vi "getBorderNum.vi"(0 "Refnum in":T1, 2 "Cut Limit":dbl format="%#_13g", 5 "Bounding Box":cluster{"x":sgl, "y":sgl}[][](array[cluster]), 7 "Position":sgl[][](array[numeric]), 9 "Angle":sgl[](array[numeric]), 11 "error in (no error)":errorcluster, 12 "Step":sgl=0.29742944, 13 "Origin Pixel":dbl[](array[numeric])) -> (4 "Refnum out":T1, 8 "Data Pieces":T3(array[cluster]) {"ROI Números"."Contours"."Type" items=["No Selection", "Point", "Line", "Rectangle", "Oval", "Polygon", "Freehand Region", "Annulus", "Unused2", "Unused3", "Broken Line", "Freehand Line", "Rotated Rectangle"]}, 15 "error out":errorcluster)   [LabVIEW 2016]
uses:
  <vilib>/vision/Image Controls.llb/IMAQ Image.ctl
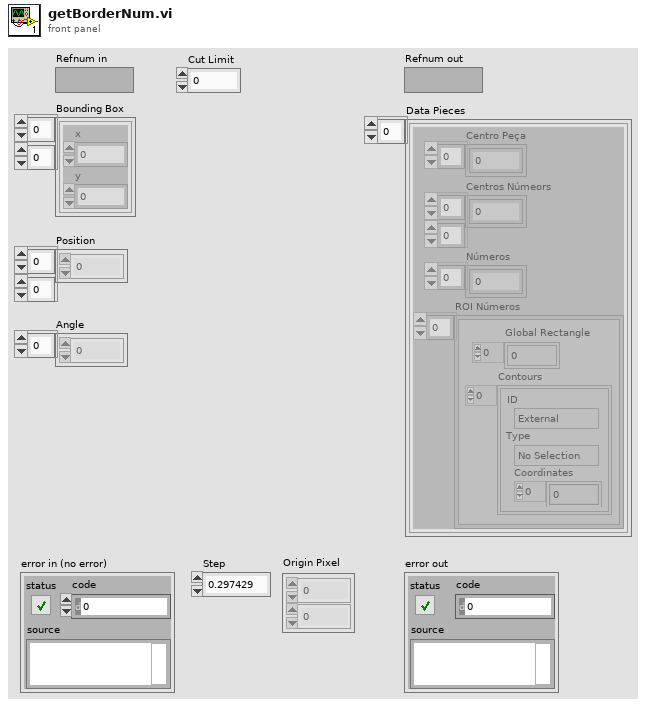
[diagram p1: front panel]
types:
  T1 = typedef "IMAQ Image.ctl" = refnum<image>
  T2 = typedef "ROI Descriptor" = cluster{"Global Rectangle":i32[], "Contours":cluster{"ID":enum32{"External", "Internal"}, "Type":u32, "Coordinates":i32[]}[]}
  T3 = cluster{"Centro Peça":dbl[], "Centros Númeors":dbl[][], "Números":u8[], "ROI Números":T2[]}[]
  T4 = cluster{"Centro Peça":dbl[], "Centros Númeors":dbl[][], "Números":u8[], "ROI Números":T2[]}
  T5 = typedef "IMAQ Rectangle" = cluster{"Left":i32, "Top":i32, "Right":i32, "Bottom":i32, "Rotation":dbl}
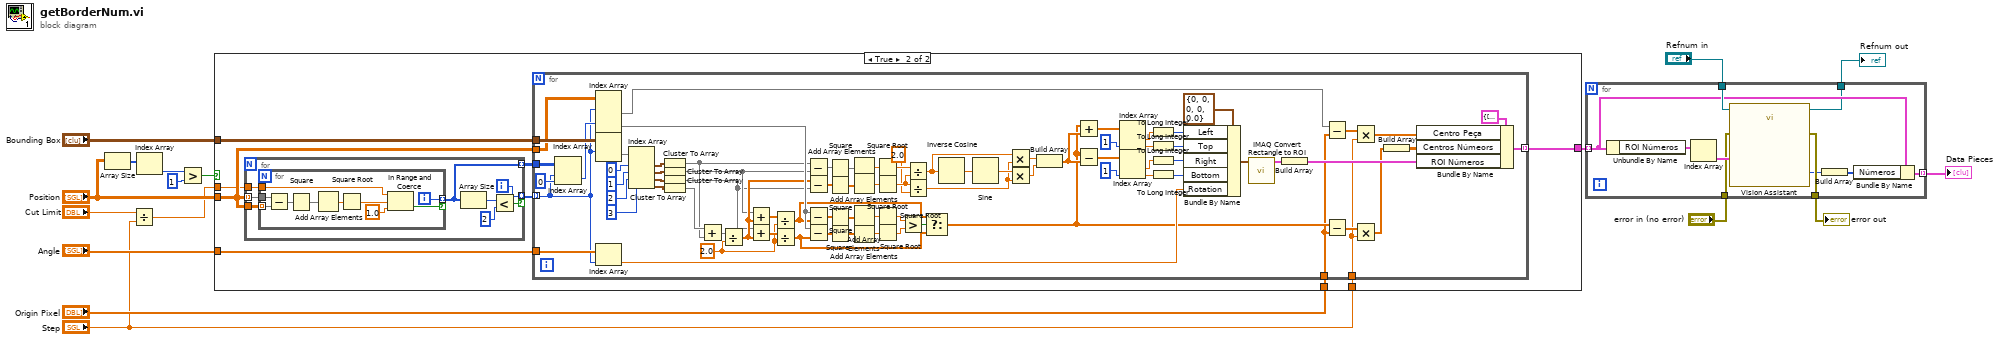
[diagram p0: block diagram]
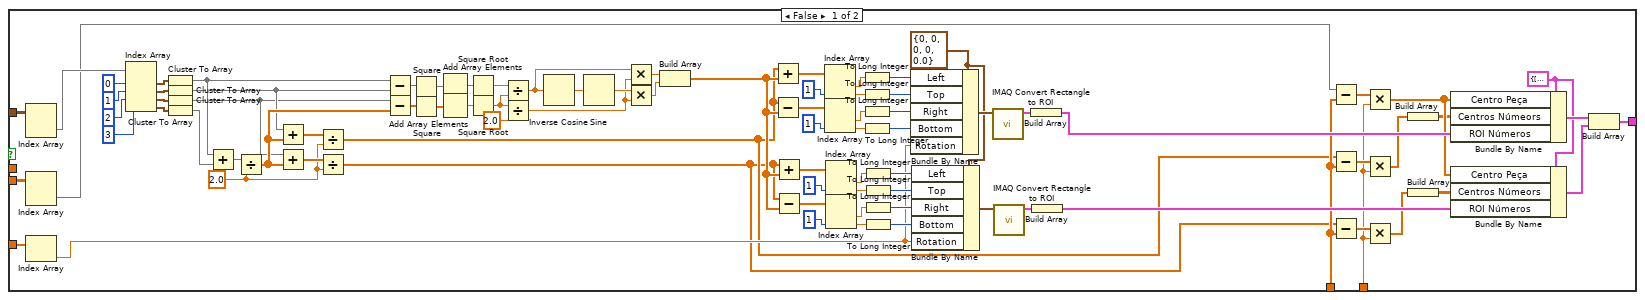
[diagram p2: hidden frame]
diagram:
  n1 = Array Size(array="Position") -> (size(s)=w7:i32[])
  n2 = Divide(x="Cut Limit", y="Step") -> (x/y=w3:dbl)
  n3 = Index Array(array=w7) -> (element=w8:i32)  [unwired: 1 in]
  n4 = Greater?(x=w8, y=1) -> (0:w6:bool)
  n5 = case shown="True" w6 {
    tunnel: "Bounding Box" -> [w103 w112]
    tunnel: "Position" -> [w102 w111]
    tunnel: "Angle" -> [w41 w109]
    tunnel: [w37 w107] -> w12
    tunnel: w3 -> [_ w106]
    tunnel: "Origin Pixel" -> [w24 w105]
    tunnel: "Step" -> [w25 w104]
    frame False {
      w36 = T4 {"Centro Peça"=[0.0, 0.0], "Centros Númeors"=[[0.0, 0.0], [0.0, 0.0]], "Números"=[0, 0], "ROI Números"=[]} ("Dados Peça")
      w42 = T5 {"Left"=0, "Top"=0, "Right"=0, "Bottom"=0, "Rotation"=0.0} ("Rectangle")
      w78 = 2.0 ("y")
      n6 = Index Array(array=w103) -> (element=w101:cluster{"x":sgl, "y":sgl}[])  [unwired: 2 in]
      n7 = Index Array(array=w102) -> (element=w29:sgl[])  [unwired: 2 in]
      n8 = Index Array(array=w41) -> (element=w40:sgl)  [unwired: 1 in]
      n9 = Index Array(array=w101, index #1=0 ("index"), index #2=1 ("index"), index #3=2 ("index"), index #4=3 ("index")) -> (element #1=w96:cluster{"x":sgl, "y":sgl}, element #2=w95:cluster{"x":sgl, "y":sgl}, element #3=w94:cluster{"x":sgl, "y":sgl}, element #4=w93:cluster{"x":sgl, "y":sgl})
      n10 = Cluster To Array(cluster=w96) -> (array=w84:sgl[])
      n11 = Cluster To Array(cluster=w95) -> (array=w82:sgl[])
      n12 = Cluster To Array(cluster=w94) -> (array=w81:sgl[])
      n13 = Cluster To Array(cluster=w93) -> (array=w89:sgl[])
      n14 = Add(x=w84, y=w89) -> (x+y=w88:sgl[])
      n15 = Divide(x=w88, y=w78) -> (x/y=w83:dbl[])
      n16 = Add(x=w82, y=w83) -> (x+y=w80:dbl[])
      n17 = Add(x=w81, y=w83) -> (x+y=w79:dbl[])
      n18 = Divide(x=w80, y=w78) -> (x/y=w23:dbl[])
      n19 = Divide(x=w79, y=w78) -> (x/y=w22:dbl[])
      n20 = Subtract(x=w84, y=w82) -> (x-y=w85:sgl[])
      n21 = Subtract(x=w81, y=w83) -> (x-y=w90:dbl[])
      n22 = Square(x=w85) -> (x^2=w87:sgl[])
      n23 = Square(x=w90) -> (x^2=w92:dbl[])
      n24 = Add Array Elements(numeric array=w87) -> (sum=w86:sgl)
      n25 = Add Array Elements(numeric array=w92) -> (sum=w91:dbl)
      n26 = Square Root(x=w86) -> (sqrt(x)=w77:sgl)
      n27 = Square Root(x=w91) -> (sqrt(x)=w76:dbl)
      n28 = Divide(x=w77, y=w76) -> (x/y=w70:dbl)
      n29 = Divide(x=w76, y=2.0) -> (x/y=w69:dbl)
      n30 = Inverse Cosine(1:w70) -> (0:w74:dbl)
      n31 = Sine(x=w74) -> (sin(x)=w73:dbl)
      n32 = Multiply(x=w70, y=w69) -> (x*y=w71:dbl)
      n33 = Multiply(x=w73, y=w69) -> (x*y=w72:dbl)
      n34 = Build Array(w71, w72) -> (w39:dbl[])
      n35 = Add(x=w23, y=w39) -> (x+y=w56:dbl[])
      n36 = Subtract(x=w23, y=w39) -> (x-y=w57:dbl[])
      n37 = Add(x=w22, y=w39) -> (x+y=w43:dbl[])
      n38 = Subtract(x=w22, y=w39) -> (x-y=w44:dbl[])
      n39 = Index Array(array=w56, index #2=1 ("index")) -> (element #1=w58:dbl, element #2=w59:dbl)  [unwired: 1 in]
      n40 = Index Array(array=w57, index #2=1 ("index")) -> (element #1=w60:dbl, element #2=w61:dbl)  [unwired: 1 in]
      n41 = Index Array(array=w43, index #2=1 ("index")) -> (element #1=w45:dbl, element #2=w46:dbl)  [unwired: 1 in]
      n42 = Index Array(array=w44, index #2=1 ("index")) -> (element #1=w47:dbl, element #2=w48:dbl)  [unwired: 1 in]
      n43 = To Long Integer(number=w58) -> (32bit integer=w65:i32)
      n44 = To Long Integer(number=w59) -> (32bit integer=w64:i32)
      n45 = To Long Integer(number=w60) -> (32bit integer=w63:i32)
      n46 = To Long Integer(number=w61) -> (32bit integer=w62:i32)
      n47 = To Long Integer(number=w45) -> (32bit integer=w52:i32)
      n48 = To Long Integer(number=w46) -> (32bit integer=w51:i32)
      n49 = To Long Integer(number=w47) -> (32bit integer=w50:i32)
      n50 = To Long Integer(number=w48) -> (32bit integer=w49:i32)
      n51 = Bundle By Name(cluster=w42, "Left"=w65, "Top"=w64, "Right"=w63, "Bottom"=w62, "Rotation"=w40) -> (w66:T5)
      n52 = Bundle By Name(cluster=w42, "Left"=w52, "Top"=w51, "Right"=w50, "Bottom"=w49, "Rotation"=w40) -> (w53:T5)
      n53 = call "IMAQ Convert Rectangle to ROI"("Rectangle"=w66) -> ("ROI Descriptor"=w35:T2)  [unwired: 8 in, 1 out]
      n54 = call "IMAQ Convert Rectangle to ROI"("Rectangle"=w53) -> ("ROI Descriptor"=w34:T2)  [unwired: 8 in, 1 out]
      n55 = Build Array(w35) -> (w32:T2[])
      n56 = Build Array(w34) -> (w33:T2[])
      n57 = Subtract(x=w29, y=w24) -> (x-y=w30:dbl[])
      n58 = Subtract(x=w23, y=w24) -> (x-y=w27:dbl[])
      n59 = Subtract(x=w22, y=w24) -> (x-y=w26:dbl[])
      n60 = Multiply(x=w30, y=w25) -> (x*y=w28:dbl[])
      n61 = Multiply(x=w27, y=w25) -> (x*y=w21:dbl[])
      n62 = Multiply(x=w26, y=w25) -> (x*y=w18:dbl[])
      n63 = Build Array(w21) -> (w20:dbl[][])
      n64 = Build Array(w18) -> (w19:dbl[][])
      n65 = Bundle By Name(cluster=w36, "Centro Peça"=w28, "Centros Númeors"=w20, "ROI Números"=w32) -> (w38:T4)
      n66 = Bundle By Name(cluster=w36, "Centro Peça"=w28, "Centros Númeors"=w19, "ROI Números"=w33) -> (w31:T4)
      n67 = Build Array(w38, w31) -> (w37:T3)
    }
    frame True {
      n68 = for {
        tunnel: w111 -> [w201] mode=indexing
        tunnel: w111 -> [w200]
        tunnel: [w199] -> w110 mode=indexing if=w196
        tunnel: [w195] -> w108 mode=indexing
        tunnel: w106 -> [w194]
        i -> [w199]
        n69 = for {
          tunnel: w201 -> [w211]
          tunnel: w200 -> [w207] mode=indexing
          tunnel: [w204] -> w195 mode=indexing if=w203
          tunnel: w194 -> [w202]
          i -> [w204]
          n70 = Subtract(x=w211, y=w207) -> (x-y=w210:sgl[])
          n71 = Square(x=w210) -> (x^2=w209:sgl[])
          n72 = Add Array Elements(numeric array=w209) -> (sum=w208:sgl)
          n73 = Square Root(x=w208) -> (sqrt(x)=w205:sgl)
          n74 = In Range and Coerce(upper limit=w202, x=w205, lower limit=1.0) -> (In Range?=w203:bool)  [unwired: 1 out]
        }
        n75 = Array Size(array=w195) -> (size(s)=w198:i32)
        n76 = Less?(x=w198, y=2) -> (x < y?=w196:bool)
      }
      n77 = for {
        tunnel: w112 -> [w193]
        tunnel: w111 -> [w191]
        tunnel: w110 -> [w153] mode=indexing
        tunnel: w109 -> [w179]
        tunnel: w108 -> [w176]
        tunnel: [w122] -> w107 mode=indexing
        tunnel: w105 -> [w114]
        tunnel: w104 -> [w113]
        w152 = 2.0 ("y")
        n78 = Index Array(array=w176, index (row)=w153, index (col)=0 ("disabled index (col)")) -> (element=w175:i32)
        n79 = Index Array(array=w191, index (row) #1=w153, index (row) #2=w175) -> (element #1=w121:sgl[], element #2=w154:sgl[])  [unwired: 2 in]
        n80 = Index Array(array=w193, index (row)=w153) -> (element=w192:cluster{"x":sgl, "y":sgl}[])  [unwired: 1 in]
        n81 = Index Array(array=w179, index=w153) -> (element=w178:sgl)
        n82 = Index Array(array=w192, index #1=0 ("index"), index #2=1 ("index"), index #3=2 ("index"), index #4=3 ("index")) -> (element #1=w189:cluster{"x":sgl, "y":sgl}, element #2=w190:cluster{"x":sgl, "y":sgl}, element #3=w188:cluster{"x":sgl, "y":sgl}, element #4=w171:cluster{"x":sgl, "y":sgl})
        n83 = Cluster To Array(cluster=w189) -> (array=w138:sgl[])
        n84 = Cluster To Array(cluster=w190) -> (array=w137:sgl[])
        n85 = Cluster To Array(cluster=w188) -> (array=w132:sgl[])
        n86 = Cluster To Array(cluster=w171) -> (array=w168:sgl[])
        n87 = Add(x=w168, y=w138) -> (x+y=w170:sgl[])
        n88 = Divide(x=w170, y=w152) -> (x/y=w143:dbl[])
        n89 = Add(x=w137, y=w143) -> (x+y=w142:dbl[])
        n90 = Add(x=w132, y=w143) -> (x+y=w167:dbl[])
        n91 = Divide(x=w142, y=w152) -> (x/y=w148:dbl[])
        n92 = Divide(x=w167, y=w152) -> (x/y=w147:dbl[])
        n93 = Subtract(x=w138, y=w137) -> (x-y=w139:sgl[])
        n94 = Subtract(x=w143, y=w132) -> (x-y=w146:dbl[])
        n95 = Subtract(x=w154, y=w148) -> (x-y=w166:dbl[])
        n96 = Subtract(x=w154, y=w147) -> (x-y=w155:dbl[])
        n97 = Square(x=w139) -> (x^2=w141:sgl[])
        n98 = Square(x=w146) -> (x^2=w144:dbl[])
        n99 = Square(x=w166) -> (x^2=w164:dbl[])
        n100 = Square(x=w155) -> (x^2=w157:dbl[])
        n101 = Add Array Elements(numeric array=w141) -> (sum=w140:sgl)
        n102 = Add Array Elements(numeric array=w144) -> (sum=w145:dbl)
        n103 = Add Array Elements(numeric array=w164) -> (sum=w165:dbl)
        n104 = Add Array Elements(numeric array=w157) -> (sum=w156:dbl)
        n105 = Square Root(x=w140) -> (sqrt(x)=w136:sgl)
        n106 = Square Root(x=w145) -> (sqrt(x)=w131:dbl)
        n107 = Square Root(x=w165) -> (sqrt(x)=w150:dbl)
        n108 = Square Root(x=w156) -> (sqrt(x)=w149:dbl)
        n109 = Greater?(x=w150, y=w149) -> (0:w151:bool)
        n110 = Divide(x=w136, y=w131) -> (x/y=w133:dbl)
        n111 = Divide(x=w131, y=2.0) -> (x/y=w129:dbl)
        n112 = Select(t=w148, s=w151, f=w147) -> (s? t:f=w115:dbl[])
        n113 = Inverse Cosine(1:w133) -> (0:w135:dbl)
        n114 = Sine(x=w135) -> (sin(x)=w134:dbl)
        n115 = Multiply(x=w133, y=w129) -> (x*y=w127:dbl)
        n116 = Multiply(x=w134, y=w129) -> (x*y=w128:dbl)
        n117 = Build Array(w127, w128) -> (w126:dbl[])
        n118 = Add(x=w115, y=w126) -> (x+y=w158:dbl[])
        n119 = Subtract(x=w115, y=w126) -> (x-y=w159:dbl[])
        n120 = Index Array(array=w158, index #2=1 ("index")) -> (element #1=w160:dbl, element #2=w161:dbl)  [unwired: 1 in]
        n121 = Index Array(array=w159, index #2=1 ("index")) -> (element #1=w162:dbl, element #2=w163:dbl)  [unwired: 1 in]
        n122 = To Long Integer(number=w160) -> (32bit integer=w183:i32)
        n123 = To Long Integer(number=w161) -> (32bit integer=w182:i32)
        n124 = To Long Integer(number=w162) -> (32bit integer=w181:i32)
        n125 = To Long Integer(number=w163) -> (32bit integer=w180:i32)
        n126 = Bundle By Name(cluster=T5 {"Left"=0, "Top"=0, "Right"=0, "Bottom"=0, "Rotation"=0.0} ("Rectangle"), "Left"=w183, "Top"=w182, "Right"=w181, "Bottom"=w180, "Rotation"=w178) -> (w184:T5)
        n127 = call "IMAQ Convert Rectangle to ROI"("Rectangle"=w184) -> ("ROI Descriptor"=w124:T2)  [unwired: 8 in, 1 out]
        n128 = Build Array(w124) -> (w123:T2[])
        n129 = Subtract(x=w121, y=w114) -> (x-y=w120:dbl[])
        n130 = Subtract(x=w115, y=w114) -> (x-y=w118:dbl[])
        n131 = Multiply(x=w120, y=w113) -> (x*y=w119:dbl[])
        n132 = Multiply(x=w118, y=w113) -> (x*y=w116:dbl[])
        n133 = Build Array(w116) -> (w117:dbl[][])
        n134 = Bundle By Name(cluster=T4 {"Centro Peça"=[0.0, 0.0], "Centros Númeors"=[[0.0, 0.0], [0.0, 0.0]], "Números"=[0, 0], "ROI Números"=[]} ("Dados Peça"), "Centro Peça"=w119, "Centros Númeors"=w117, "ROI Números"=w123) -> (w122:T4)
      }
    }
  }
  n135 = for {
    tunnel: w12 -> [w217] mode=indexing
    tunnel: "Refnum in" -> [w219]
    tunnel: [w218] -> w13
    tunnel: [w214] -> w14 mode=indexing
    tunnel: "error in (no error)" -> [w213]
    tunnel: [w212] -> w5
    n136 = Unbundle By Name(w217) -> ("ROI Números"=w221:T2[])
    n137 = Index Array(array=w221) -> (element=w220:T2)  [unwired: 1 in]
    n138 = call "Vision Assistant"("Image In"=w219, "ROI Descriptor (Image Mask 1)"=w220, "error in"=w213) -> ("Image Out"=w212:T1, "Number of Particles (Particle Analysis 1)"=w216:i32, "error out"=w218:errorcluster)  [unwired: 22 in]
    n139 = Build Array(w216) -> (w215:i32[])
    n140 = Bundle By Name(cluster=w217, "Números"=w215) -> (w214:T4)
  }
  "Data Pieces" <- w14
  "error out" <- w13
  "Refnum out" <- w5
